vi "MPExxx_get_ocp.vi"(0 "VISA session":refnum<visa-resource-name>, 1 "error in (no error)":errorcluster) -> (2 "dup VISA session":refnum<visa-resource-name>, 3 "OCP Setting":string, 4 "error out":errorcluster)   [LabVIEW 2012]
doc: "This VI form retrieves the over current trip level of the power supply."
panel:
  # "MAGNA-POWER"
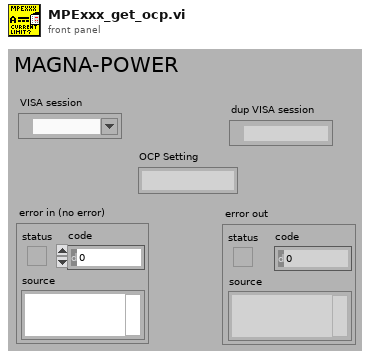
[diagram p1: front panel]
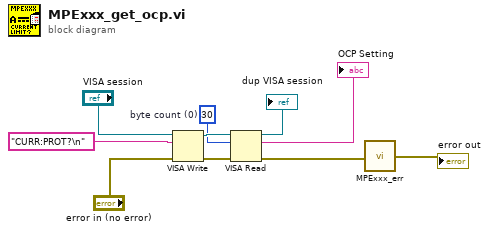
[diagram p0: block diagram]
diagram:
  w8 = u32 30  # byte count (0)
  n1 = VISA Write(VISA resource name="VISA session", write buffer="CURR:PROT?\n", error in (no error)="error in (no error)") -> (VISA resource name out=w9:refnum<visa-resource-name>, error out=w7:errorcluster)  [unwired: 1 out]
  n2 = VISA Read(VISA resource name=w9, byte count=w8, error in (no error)=w7) -> (VISA resource name out=→"dup VISA session":refnum<visa-resource-name>, read buffer=→"OCP Setting":string, error out=w2:errorcluster)  [unwired: 1 out]
  n3 = call "MPExxx_err.vi"("error in (no error)"=w2) -> ("error out"=→"error out":errorcluster)
